vi "Display Continuous Probability Distributions.vi"() -> ()   [LabVIEW 2023]
doc: "This example VI uses Continuous PDF.vi, Continuous CDF.vi, Continuous Inverse CDF.vi to display continuous probability density functions, cumulative distribution functions, and inverse cumulative distribution functions for the beta, cauchy, chi-squared, exponential, gamma, laplace, and normal distributions."
uses:
  <vilib>/Analysis/1siggen.llb/Ramp Pattern by Samples.vi
  <vilib>/gmath/statdist.llb/Normal Moments.vi
  <vilib>/gmath/statdist.llb/Normal CDF.vi
  <vilib>/gmath/statdist.llb/Normal Inverse CDF.vi
  <vilib>/gmath/statdist.llb/Normal PDF.vi
  <vilib>/gmath/statdist.llb/Uniform CDF.vi
  <vilib>/gmath/statdist.llb/Uniform Inverse CDF.vi
  <vilib>/gmath/statdist.llb/Uniform PDF.vi
  <vilib>/gmath/statdist.llb/Uniform Moments.vi
  <vilib>/gmath/statdist.llb/Beta Moments.vi
  <vilib>/gmath/statdist.llb/Beta CDF.vi
  <vilib>/gmath/statdist.llb/Beta Inverse CDF.vi
  <vilib>/gmath/statdist.llb/Beta PDF.vi
  <vilib>/gmath/statdist.llb/Cauchy CDF.vi
  <vilib>/gmath/statdist.llb/Cauchy Inverse CDF.vi
  <vilib>/gmath/statdist.llb/Cauchy PDF.vi
  <vilib>/gmath/statdist.llb/Chi-Squared Moments.vi
  <vilib>/gmath/statdist.llb/Chi-Squared CDF.vi
  <vilib>/gmath/statdist.llb/Chi-Squared Inverse CDF.vi
  <vilib>/gmath/statdist.llb/Chi-Squared PDF.vi
  <vilib>/gmath/statdist.llb/Exp Moments.vi
  <vilib>/gmath/statdist.llb/Exp CDF.vi
  <vilib>/gmath/statdist.llb/Exp Inverse CDF.vi
  <vilib>/gmath/statdist.llb/Exp PDF.vi
  <vilib>/gmath/statdist.llb/Lognormal CDF.vi
  <vilib>/gmath/statdist.llb/Lognormal Inverse CDF.vi
  <vilib>/gmath/statdist.llb/Lognormal PDF.vi
  <vilib>/gmath/statdist.llb/Lognormal Moments.vi
  <vilib>/gmath/statdist.llb/Gamma Moments.vi
  <vilib>/gmath/statdist.llb/Gamma CDF.vi
  <vilib>/gmath/statdist.llb/Gamma Inverse CDF.vi
  <vilib>/gmath/statdist.llb/Gamma PDF.vi
  <vilib>/gmath/statdist.llb/Laplace Moments.vi
  <vilib>/gmath/statdist.llb/Laplace CDF.vi
  <vilib>/gmath/statdist.llb/Laplace Inverse CDF.vi
  <vilib>/gmath/statdist.llb/Laplace PDF.vi
  <vilib>/gmath/NI_Gmath.lvlib
  <vilib>/Analysis/NI_AALBase.lvlib
panel:
  in  "Stop":bool
  in  "Tab Control":T1(tab)
  in  "std (Normal)":dbl(slide)=4.0 min=0.0 scale=0.5..4.0
  in  "mean (Normal)":dbl(slide) scale=-5.0..5.0
  in  "end (Normal)":dbl=15.0
  in  "start (Normal)":dbl=-15.0
  in  "samples (Normal)":i32=200
  out "Variance (Normal)":dbl
  out "Mean (Normal)":dbl
  out "Normal Inverse Cumulative Distribution Function":cluster{dbl[], dbl[]}(graph)
  out "Normal Cumulative Distribution Function":cluster{"Ramp Pattern":dbl[], dbl[]}(graph)
  out "Normal Probability Density Function":cluster{"Ramp Pattern":dbl[], dbl[]}(graph)
  in  "x max":dbl(slide)=5.0 min=0.0 scale=0.0..5.0
  in  "x min":dbl(slide)=-5.0
  in  "end (Uniform)":dbl=10.0
  in  "start (Uniform)":dbl=-10.0
  in  "samples (Uniform)":i32=200
  out "Variance (Uniform)":dbl
  out "Mean (Uniform)":dbl
  out "Uniform Inverse Cumulative Distribution Function":cluster{dbl[], dbl[]}(graph)
  out "Uniform Cumulative Distribution Function":cluster{"Ramp Pattern":dbl[], dbl[]}(graph)
  out "Uniform Probability Density Function":cluster{"Ramp Pattern":dbl[], dbl[]}(graph)
  in  "start (Beta)":dbl min=0.0 max=1.0
  in  "end (Beta)":dbl=1.0 min=0.0 max=1.0
  in  "samples (Beta)":i32=100
  out "Variance (Beta)":dbl=0.031746031746031744
  out "Mean (Beta)":dbl=0.3333333333333333
  in  "b (Beta)":dbl(slide)=4.0 min=0.0 scale=0.1..100.0
  in  "a (Beta)":dbl(slide)=2.0 min=0.0 scale=0.1..10.0
  out "Beta Inverse Cumulative Distribution Function":cluster{dbl[], dbl[]}(graph)
  out "Beta Cumulative Distribution Function":cluster{"Ramp Pattern":dbl[], dbl[]}(graph)
  out "Beta Probability Density Function":cluster{"Ramp Pattern":dbl[], dbl[]}(graph)
  in  "end (Cauchy)":dbl=10.0
  in  "samples (Cauchy)":i32=100
  in  "start (Cauchy)":dbl=-10.0
  in  "b (Cauchy)":dbl(slide)=1.0 min=0.0 scale=0.1..10.0
  in  "a (Cauchy)":dbl(slide) scale=-10.0..10.0
  out "Cauchy Inverse Cumulative Distribution Function":cluster{dbl[], dbl[]}(graph)
  out "Cauchy Cumulative Distribution Function":cluster{"Ramp Pattern":dbl[], dbl[]}(graph)
  out "Cauchy Probability Density Function":cluster{"Ramp Pattern":dbl[], dbl[]}(graph)
  in  "end (Chi-Squared)":dbl=200.0
  in  "start (Chi-Squared)":dbl min=0.0
  in  "samples (Chi-Squared)":i32=200
  out "Variance (Chi-Squared)":dbl
  out "Mean (Chi-Squared)":dbl
  in  "degrees of freedom (k)":i32(slide)=80 min=1 scale=1.0..40.0
  out "Chi-Square Inverse Cumulative Distribution Function":cluster{dbl[], dbl[]}(graph)
  out "Chi-Square Cumulative Distribution Function":cluster{"Ramp Pattern":dbl[], dbl[]}(graph)
  out "Chi-Square Probability Density Function":cluster{"Ramp Pattern":dbl[], dbl[]}(graph)
  out "Exponential Cumulative Distribution Function":cluster{"Ramp Pattern":dbl[], dbl[]}(graph)
  in  "end (Exp)":dbl=15.0
  in  "start (Exp)":dbl min=0.0
  in  "samples (Exp)":i32=100
  out "Variance (Exp)":dbl
  out "Mean (Exp)":dbl
  in  "b (Exp)":dbl(slide)=4.0 min=0.0 scale=0.1..10.0
  in  "a (Exp)":dbl(slide) scale=0.0..10.0
  out "Exponential Inverse Cumulative Distribution Function":cluster{dbl[], dbl[]}(graph)
  out "Exponential Probability Density Function":cluster{"Ramp Pattern":dbl[], dbl[]}(graph)
  in  "location type":enum16{"mu - mean (log(X))", "median (X)"}(ring)
  in  "samples (Lognormal)":i32=200
  in  "mu or median (Lognormal)":dbl(slide)=1.0 scale=-5.0..5.0
  in  "start (Lognormal)":dbl
  in  "end (Lognormal)":dbl=10.0
  in  "std (Lognormal)":dbl(slide)=1.0 min=0.0 scale=0.5..4.0
  out "Variance (Lognormal)":dbl
  out "Mean (Lognormal)":dbl
  out "Lognormal Cumulative Distribution Function":cluster{"Ramp Pattern":dbl[], dbl[]}(graph)
  out "Lognormal Inverse Cumulative Distribution Function":cluster{dbl[], dbl[]}(graph)
  out "Lognormal PDF":cluster{"Ramp Pattern":dbl[], dbl[]}(graph)
  in  "end (Gamma)":dbl=100.0
  in  "start (Gamma)":dbl min=0.0
  in  "samples (Gamma)":i32=200
  out "Variance (Gamma)":dbl
  out "Mean (Gamma)":dbl
  in  "c (Gamma)":dbl(slide)=7.0 min=0.0 scale=0.1..10.0
  in  "b (Gamma)":dbl(slide)=3.0 min=0.0 scale=1.0..10.0
  out "Gamma Inverse Cumulative Distribution Function":cluster{dbl[], dbl[]}(graph)
  out "Gamma Cumulative Distribution Function":cluster{"Ramp Pattern":dbl[], dbl[]}(graph)
  out "Gamma Probability Density Function":cluster{"Ramp Pattern":dbl[], dbl[]}(graph)
  in  "end (Laplace)":dbl=15.0
  in  "start (Laplace)":dbl=-15.0
  in  "samples (Laplace)":i32=200
  in  "b (Laplace)":dbl(slide)=3.0 min=0.0 scale=0.0..10.0
  in  "a (Laplace)":dbl(slide) scale=-5.0..5.0
  out "Variance (Laplace)":dbl
  out "Mean (Laplace)":dbl
  out "Laplace Inverse Cumulative Distribution Function":cluster{dbl[], dbl[]}(graph)
  out "Laplace Cumulative Distribution Function":cluster{"Ramp Pattern":dbl[], dbl[]}(graph)
  out "Laplace Probability Density Function":cluster{"Ramp Pattern":dbl[], dbl[]}(graph)
  # "Overview: Demonstrates the use of the Continuous PDF VI, Continuous CDF VI, and Continuous Inverse CDF VI.\nInstructions:\n1. Run the VI.\n2. Switch between tabs to explore how the parameters affect each distribution.\n3. Click Stop to stop the VI."
  # "NOTE: According to theory, the Cauchy distribution does not have a moment generating function (mean and variance)"
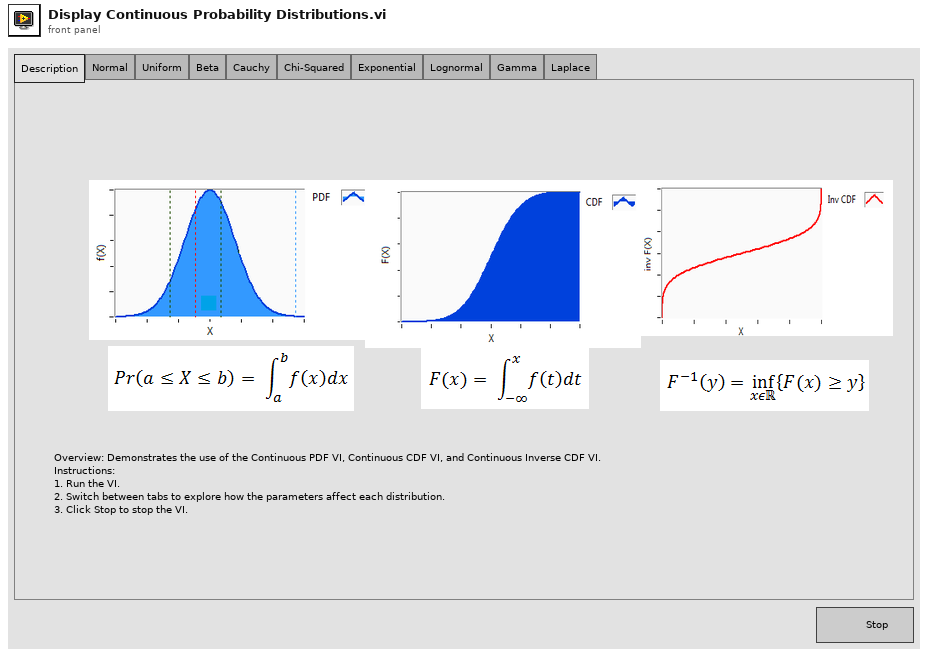
[diagram p1: front panel]
types:
  T1 = enum32{"Description", "Normal", "Uniform", "Beta", "Cauchy", "Chi-Squared", "Exponential", "Lognormal", "Gamma", "Laplace"}
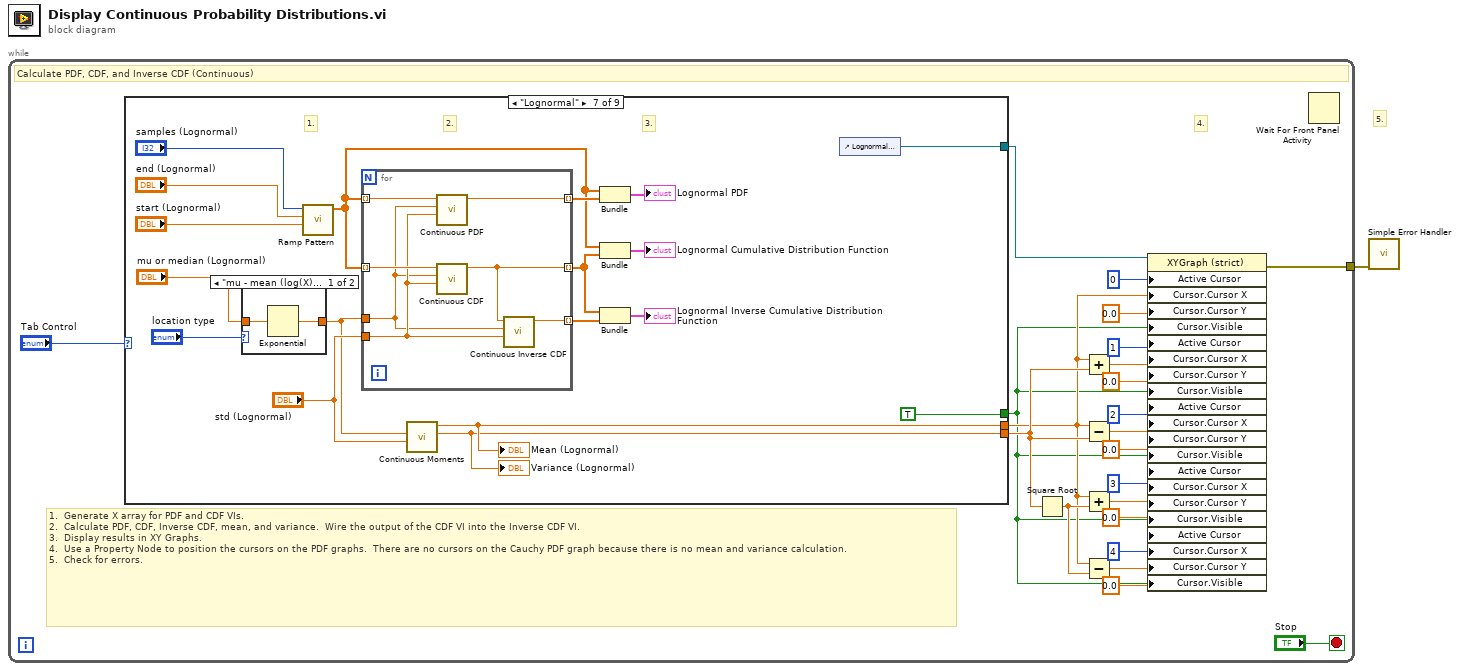
[diagram p0: block diagram]
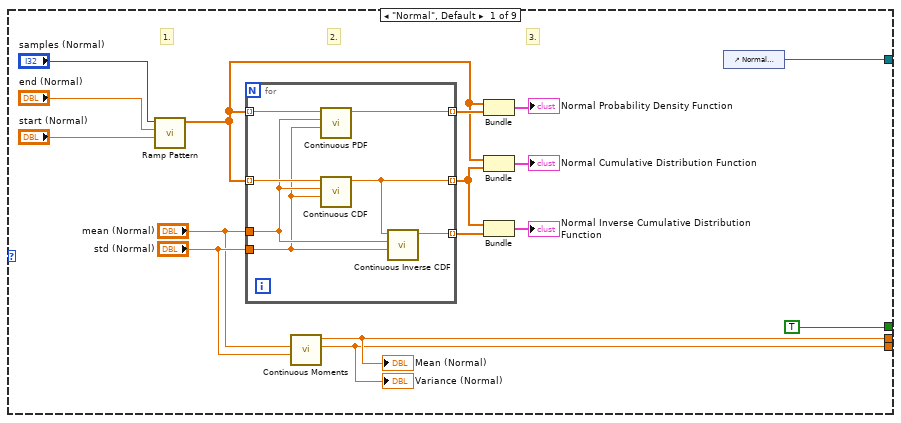
[diagram p2: hidden frame]
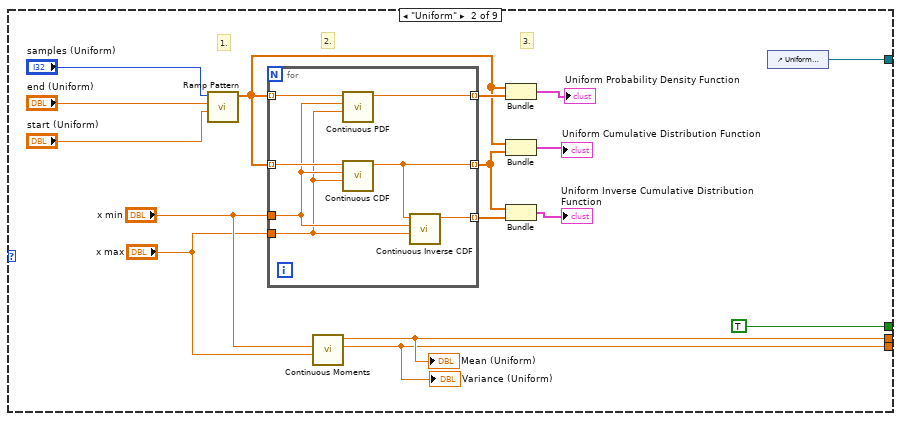
[diagram p3: hidden frame]
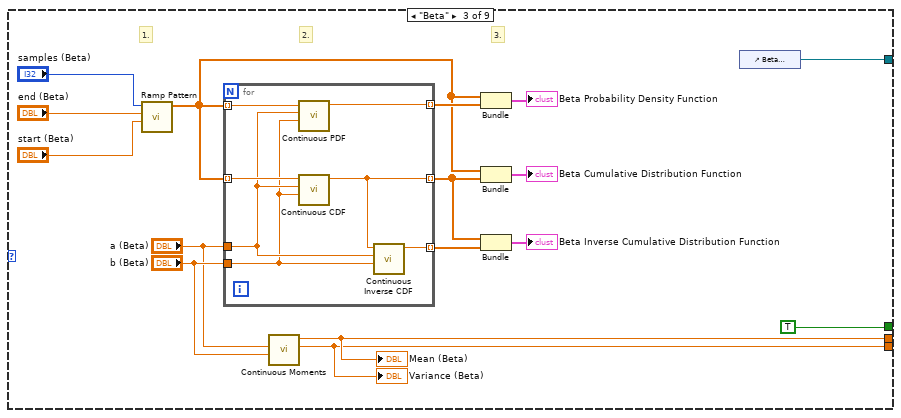
[diagram p4: hidden frame]
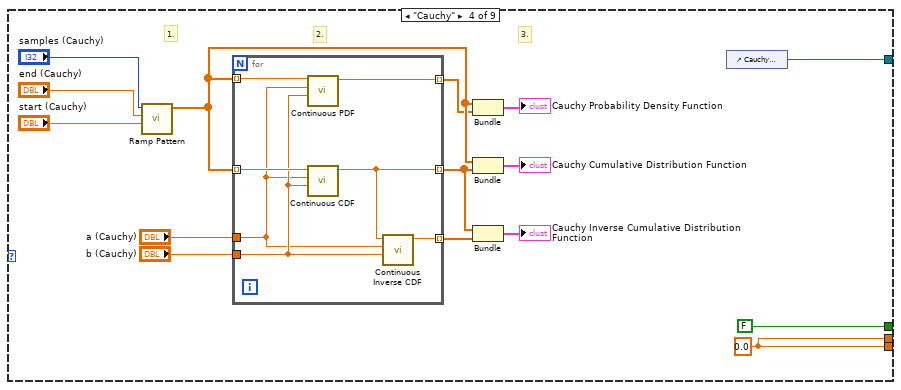
[diagram p5: hidden frame]
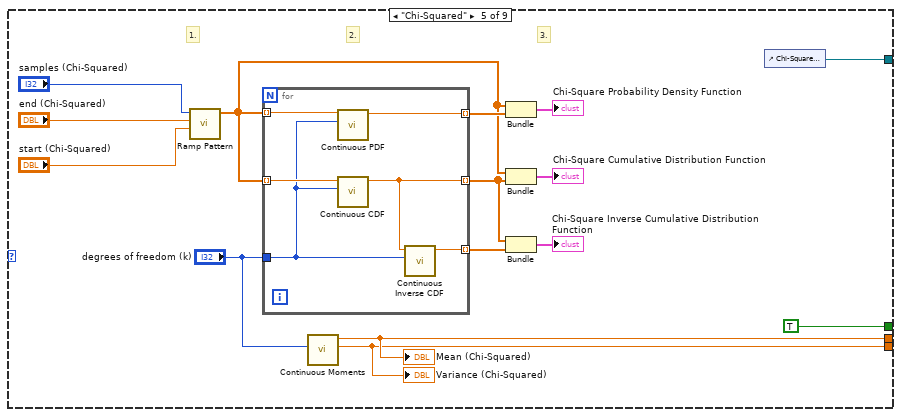
[diagram p6: hidden frame]
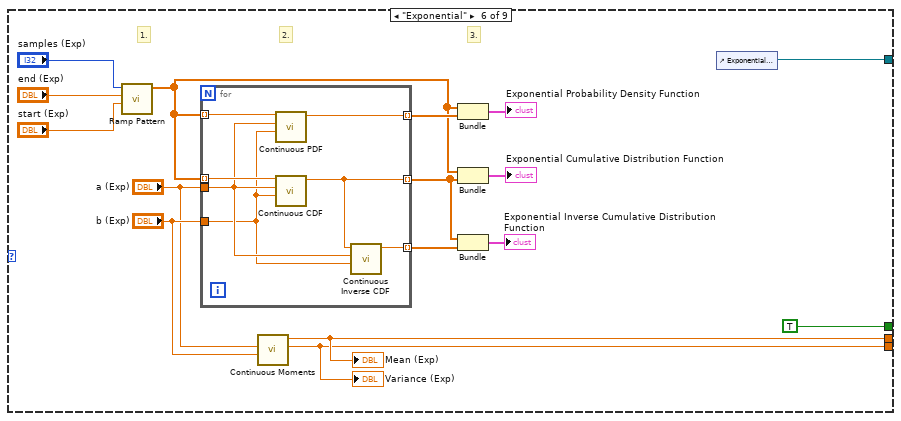
[diagram p7: hidden frame]
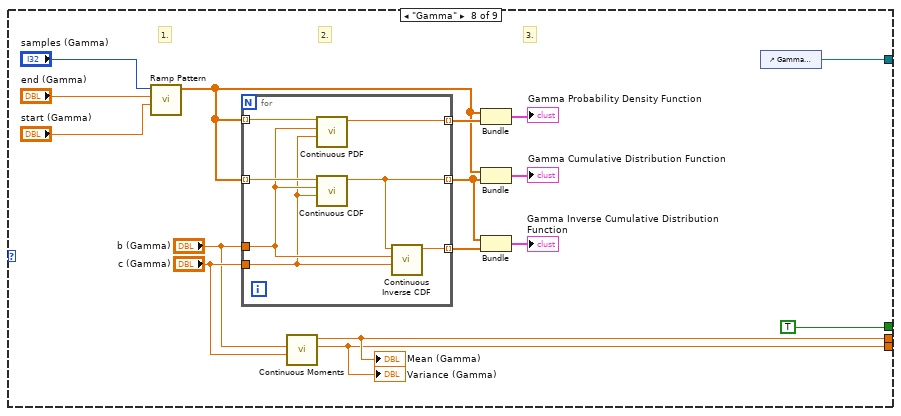
[diagram p9: hidden frame]
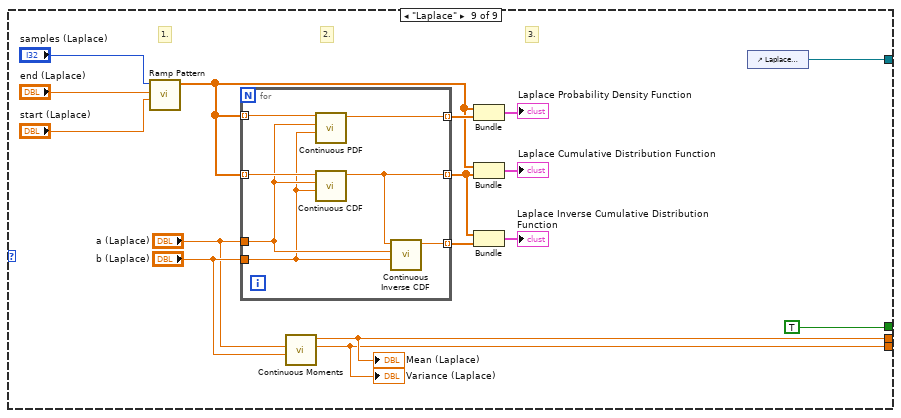
[diagram p10: hidden frame]
diagram:
  # "5."
  n1 = while {
    tunnel: [w5] -> w1
    stop <- "Stop" stop-if-true
    # "1.  Generate X array for PDF and CDF VIs.\n2.  Calculate PDF, CDF, Inverse CDF, mean, and variance.  Wire the output of the CDF VI into the Inverse CDF VI.  \n3.  Display results in XY Graphs.\n4.  Use a Property Node to position the cursors on the PDF graphs.  There are no cursors on the Cauchy PDF graph because there is no mean and variance calculation.\n5.  Check for errors."
    # "4."
    # "Calculate PDF, CDF, and Inverse CDF (Continuous)"
    n2 = case shown="\"Lognormal\"" "Tab Control" {
      tunnel: [w27 w53 w73 w94 w119 w139 w165 w190 w213] -> w4
      tunnel: [w26 w50 w72 w93 w118 w138 w164 w189 w212] -> w3
      tunnel: [w25 w49 w71 w93 w117 w137 w163 w188 w211] -> w10
      tunnel: [TRUE TRUE TRUE FALSE TRUE TRUE TRUE TRUE TRUE] -> w2
      frame "Normal", Default {
        # "3."
        # "2."
        # "1."
        n3 = call-poly <vilib>:"Ramp Pattern.vi"("start"="start (Normal)", "end"="end (Normal)", "samples"="samples (Normal)") -> ("Ramp Pattern"=w35:dbl[])  [unwired: 7 in, 1 out]
        n4 = for {
          tunnel: w35 -> [w46] mode=indexing
          tunnel: [w45] -> w36 mode=indexing
          tunnel: w35 -> [w44] mode=indexing
          tunnel: [w43] -> w33 mode=indexing
          tunnel: [w42] -> w34 mode=indexing
          tunnel: "mean (Normal)" -> [w41]
          tunnel: "std (Normal)" -> [w40]
          n5 = call-poly <vilib>:"Continuous PDF.vi"("std"=w40, "mean"=w41, "x"=w46) -> ("pdf(x)"=w45:dbl)  [unwired: 7 in, 1 out]
          n6 = call-poly <vilib>:"Continuous CDF.vi"("std"=w40, "mean"=w41, "x"=w44) -> ("cdf(x)"=w43:dbl)  [unwired: 7 in, 1 out]
          n7 = call-poly <vilib>:"Continuous Inverse CDF.vi"("std"=w40, "mean"=w41, "cdf(x)"=w43) -> ("x"=w42:dbl)  [unwired: 7 in, 1 out]
        }
        n8 = call-poly <vilib>:"Continuous Moments.vi"("std"="std (Normal)", "mean"="mean (Normal)") -> ("variance"=w25:dbl, "mean"=w26:dbl)  [unwired: 7 in, 1 out]
        "Mean (Normal)" <- w26
        "Variance (Normal)" <- w25
        n9 = Bundle("Ramp Pattern"=w35, w36) -> (→"Normal Probability Density Function":cluster{"Ramp Pattern":dbl[], dbl[]})  [unwired: 1 in]
        n10 = Bundle("Ramp Pattern"=w35, w33) -> (→"Normal Cumulative Distribution Function":cluster{"Ramp Pattern":dbl[], dbl[]})  [unwired: 1 in]
        n11 = Bundle(w33, w34) -> (→"Normal Inverse Cumulative Distribution Function":cluster{dbl[], dbl[]})  [unwired: 1 in]
        n12 = control-ref of="Normal Probability Density Function"() -> (w27:refnum<vi>)
      }
      frame "Uniform" {
        # "3."
        # "2."
        # "1."
        n13 = call-poly <vilib>:"Ramp Pattern.vi"("start"="start (Uniform)", "end"="end (Uniform)", "samples"="samples (Uniform)") -> ("Ramp Pattern"=w61:dbl[])  [unwired: 7 in, 1 out]
        n14 = for {
          tunnel: w61 -> [w69] mode=indexing
          tunnel: [w68] -> w62 mode=indexing
          tunnel: w61 -> [w67] mode=indexing
          tunnel: [w66] -> w59 mode=indexing
          tunnel: [w65] -> w60 mode=indexing
          tunnel: "x min" -> [w64]
          tunnel: "x max" -> [w63]
          n15 = call-poly <vilib>:"Continuous PDF.vi"("xmax"=w63, "xmin"=w64, "x"=w69) -> ("pdf(x)"=w68:dbl)  [unwired: 7 in, 1 out]
          n16 = call-poly <vilib>:"Continuous CDF.vi"("xmax"=w63, "xmin"=w64, "x"=w67) -> ("cdf(x)"=w66:dbl)  [unwired: 7 in, 1 out]
          n17 = call-poly <vilib>:"Continuous Inverse CDF.vi"("xmax"=w63, "xmin"=w64, "cdf(x)"=w66) -> ("x"=w65:dbl)  [unwired: 7 in, 1 out]
        }
        n18 = call-poly <vilib>:"Continuous Moments.vi"("xmax"="x max", "xmin"="x min") -> ("variance"=w49:dbl, "mean"=w50:dbl)  [unwired: 7 in, 1 out]
        "Mean (Uniform)" <- w50
        "Variance (Uniform)" <- w49
        n19 = Bundle("Ramp Pattern"=w61, w62) -> (→"Uniform Probability Density Function":cluster{"Ramp Pattern":dbl[], dbl[]})  [unwired: 1 in]
        n20 = Bundle("Ramp Pattern"=w61, w59) -> (→"Uniform Cumulative Distribution Function":cluster{"Ramp Pattern":dbl[], dbl[]})  [unwired: 1 in]
        n21 = Bundle(w59, w60) -> (→"Uniform Inverse Cumulative Distribution Function":cluster{dbl[], dbl[]})  [unwired: 1 in]
        n22 = control-ref of="Uniform Probability Density Function"() -> (w53:refnum<vi>)
      }
      frame "Beta" {
        # "3."
        # "2."
        # "1."
        n23 = call-poly <vilib>:"Ramp Pattern.vi"("start"="start (Beta)", "end"="end (Beta)", "samples"="samples (Beta)") -> ("Ramp Pattern"=w81:dbl[])  [unwired: 7 in, 1 out]
        n24 = for {
          tunnel: w81 -> [w92] mode=indexing
          tunnel: [w91] -> w82 mode=indexing
          tunnel: w81 -> [w90] mode=indexing
          tunnel: [w89] -> w79 mode=indexing
          tunnel: [w88] -> w80 mode=indexing
          tunnel: "a (Beta)" -> [w87]
          tunnel: "b (Beta)" -> [w86]
          n25 = call-poly <vilib>:"Continuous PDF.vi"("b"=w86, "a"=w87, "x"=w92) -> ("pdf(x)"=w91:dbl)  [unwired: 7 in, 1 out]
          n26 = call-poly <vilib>:"Continuous CDF.vi"("b"=w86, "a"=w87, "x"=w90) -> ("cdf(x)"=w89:dbl)  [unwired: 7 in, 1 out]
          n27 = call-poly <vilib>:"Continuous Inverse CDF.vi"("b"=w86, "a"=w87, "cdf(x)"=w89) -> ("x"=w88:dbl)  [unwired: 7 in, 1 out]
        }
        n28 = call-poly <vilib>:"Continuous Moments.vi"("b"="b (Beta)", "a"="a (Beta)") -> ("variance"=w71:dbl, "mean"=w72:dbl)  [unwired: 7 in, 1 out]
        "Mean (Beta)" <- w72
        "Variance (Beta)" <- w71
        n29 = Bundle("Ramp Pattern"=w81, w82) -> (→"Beta Probability Density Function":cluster{"Ramp Pattern":dbl[], dbl[]})  [unwired: 1 in]
        n30 = Bundle("Ramp Pattern"=w81, w79) -> (→"Beta Cumulative Distribution Function":cluster{"Ramp Pattern":dbl[], dbl[]})  [unwired: 1 in]
        n31 = Bundle(w79, w80) -> (→"Beta Inverse Cumulative Distribution Function":cluster{dbl[], dbl[]})  [unwired: 1 in]
        n32 = control-ref of="Beta Probability Density Function"() -> (w73:refnum<vi>)
      }
      frame "Cauchy" {
        w93 = 0.0
        # "3."
        # "2."
        # "1."
        n33 = call-poly <vilib>:"Ramp Pattern.vi"("start"="start (Cauchy)", "end"="end (Cauchy)", "samples"="samples (Cauchy)") -> ("Ramp Pattern"=w100:dbl[])  [unwired: 7 in, 1 out]
        n34 = for {
          tunnel: w100 -> [w114] mode=indexing
          tunnel: [w113] -> w99 mode=indexing
          tunnel: w100 -> [w112] mode=indexing
          tunnel: [w111] -> w104 mode=indexing
          tunnel: [w110] -> w105 mode=indexing
          tunnel: "a (Cauchy)" -> [w108]
          tunnel: "b (Cauchy)" -> [w109]
          n35 = call-poly <vilib>:"Continuous PDF.vi"("b"=w109, "a"=w108, "x"=w114) -> ("pdf(x)"=w113:dbl)  [unwired: 7 in, 1 out]
          n36 = call-poly <vilib>:"Continuous CDF.vi"("b"=w109, "a"=w108, "x"=w112) -> ("cdf(x)"=w111:dbl)  [unwired: 7 in, 1 out]
          n37 = call-poly <vilib>:"Continuous Inverse CDF.vi"("b"=w109, "a"=w108, "cdf(x)"=w111) -> ("x"=w110:dbl)  [unwired: 7 in, 1 out]
        }
        n38 = Bundle("Ramp Pattern"=w100, w99) -> (→"Cauchy Probability Density Function":cluster{"Ramp Pattern":dbl[], dbl[]})  [unwired: 1 in]
        n39 = Bundle("Ramp Pattern"=w100, w104) -> (→"Cauchy Cumulative Distribution Function":cluster{"Ramp Pattern":dbl[], dbl[]})  [unwired: 1 in]
        n40 = Bundle(w104, w105) -> (→"Cauchy Inverse Cumulative Distribution Function":cluster{dbl[], dbl[]})  [unwired: 1 in]
        n41 = control-ref of="Cauchy Probability Density Function"() -> (w94:refnum<vi>)
      }
      frame "Chi-Squared" {
        # "3."
        # "2."
        # "1."
        n42 = call-poly <vilib>:"Ramp Pattern.vi"("start"="start (Chi-Squared)", "end"="end (Chi-Squared)", "samples"="samples (Chi-Squared)") -> ("Ramp Pattern"=w126:dbl[])  [unwired: 7 in, 1 out]
        n43 = for {
          tunnel: w126 -> [w135] mode=indexing
          tunnel: [w134] -> w127 mode=indexing
          tunnel: w126 -> [w133] mode=indexing
          tunnel: [w132] -> w124 mode=indexing
          tunnel: [w131] -> w125 mode=indexing
          tunnel: "degrees of freedom (k)" -> [w130]
          n44 = call-poly <vilib>:"Continuous PDF.vi"("k"=w130, "x"=w135) -> ("pdf(x)"=w134:dbl)  [unwired: 8 in, 1 out]
          n45 = call-poly <vilib>:"Continuous CDF.vi"("k"=w130, "x"=w133) -> ("cdf(x)"=w132:dbl)  [unwired: 8 in, 1 out]
          n46 = call-poly <vilib>:"Continuous Inverse CDF.vi"("k"=w130, "cdf(x)"=w132) -> ("x"=w131:dbl)  [unwired: 8 in, 1 out]
        }
        n47 = call-poly <vilib>:"Continuous Moments.vi"("k"="degrees of freedom (k)") -> ("variance"=w117:dbl, "mean"=w118:dbl)  [unwired: 8 in, 1 out]
        "Mean (Chi-Squared)" <- w118
        "Variance (Chi-Squared)" <- w117
        n48 = Bundle("Ramp Pattern"=w126, w127) -> (→"Chi-Square Probability Density Function":cluster{"Ramp Pattern":dbl[], dbl[]})  [unwired: 1 in]
        n49 = Bundle("Ramp Pattern"=w126, w124) -> (→"Chi-Square Cumulative Distribution Function":cluster{"Ramp Pattern":dbl[], dbl[]})  [unwired: 1 in]
        n50 = Bundle(w124, w125) -> (→"Chi-Square Inverse Cumulative Distribution Function":cluster{dbl[], dbl[]})  [unwired: 1 in]
        n51 = control-ref of="Chi-Square Probability Density Function"() -> (w119:refnum<vi>)
      }
      frame "Exponential" {
        # "3."
        # "2."
        # "1."
        n52 = call-poly <vilib>:"Ramp Pattern.vi"("start"="start (Exp)", "end"="end (Exp)", "samples"="samples (Exp)") -> ("Ramp Pattern"=w147:dbl[])  [unwired: 7 in, 1 out]
        n53 = for {
          tunnel: w147 -> [w158] mode=indexing
          tunnel: [w157] -> w148 mode=indexing
          tunnel: w147 -> [w156] mode=indexing
          tunnel: [w155] -> w145 mode=indexing
          tunnel: [w154] -> w146 mode=indexing
          tunnel: "a (Exp)" -> [w153]
          tunnel: "b (Exp)" -> [w152]
          n54 = call-poly <vilib>:"Continuous PDF.vi"("b"=w152, "a"=w153, "x"=w158) -> ("pdf(x)"=w157:dbl)  [unwired: 7 in, 1 out]
          n55 = call-poly <vilib>:"Continuous CDF.vi"("b"=w152, "a"=w153, "x"=w156) -> ("cdf(x)"=w155:dbl)  [unwired: 7 in, 1 out]
          n56 = call-poly <vilib>:"Continuous Inverse CDF.vi"("b"=w152, "a"=w153, "cdf(x)"=w155) -> ("x"=w154:dbl)  [unwired: 7 in, 1 out]
        }
        n57 = call-poly <vilib>:"Continuous Moments.vi"("b"="b (Exp)", "a"="a (Exp)") -> ("variance"=w137:dbl, "mean"=w138:dbl)  [unwired: 7 in, 1 out]
        "Mean (Exp)" <- w138
        "Variance (Exp)" <- w137
        n58 = Bundle("Ramp Pattern"=w147, w148) -> (→"Exponential Probability Density Function":cluster{"Ramp Pattern":dbl[], dbl[]})  [unwired: 1 in]
        n59 = Bundle("Ramp Pattern"=w147, w145) -> (→"Exponential Cumulative Distribution Function":cluster{"Ramp Pattern":dbl[], dbl[]})  [unwired: 1 in]
        n60 = Bundle(w145, w146) -> (→"Exponential Inverse Cumulative Distribution Function":cluster{dbl[], dbl[]})  [unwired: 1 in]
        n61 = control-ref of="Exponential Probability Density Function"() -> (w139:refnum<vi>)
      }
      frame "Lognormal" {
        # "3."
        # "2."
        # "1."
        n62 = case shown="\"mu - mean (log(X))\", Default" "location type" {
          tunnel: "mu or median (Lognormal)" -> [w178 w179]
          tunnel: [w177 w179] -> w160
          frame "mu - mean (log(X))", Default {
            n63 = Exponential(1:w178) -> (0:w177:dbl)
          }
          frame "median (X)" {
          }
        }
        n64 = call-poly <vilib>:"Ramp Pattern.vi"("start"="start (Lognormal)", "end"="end (Lognormal)", "samples"="samples (Lognormal)") -> ("Ramp Pattern"=w172:dbl[])  [unwired: 7 in, 1 out]
        n65 = for {
          tunnel: w172 -> [w186] mode=indexing
          tunnel: [w185] -> w173 mode=indexing
          tunnel: w172 -> [w184] mode=indexing
          tunnel: [w183] -> w170 mode=indexing
          tunnel: [w182] -> w171 mode=indexing
          tunnel: w160 -> [w180]
          tunnel: "std (Lognormal)" -> [w181]
          n66 = call-poly <vilib>:"Continuous PDF.vi"("c"=w181, "b"=w180, "x"=w186) -> ("pdf(x)"=w185:dbl)  [unwired: 7 in, 1 out]
          n67 = call-poly <vilib>:"Continuous CDF.vi"("c"=w181, "b"=w180, "x"=w184) -> ("cdf(x)"=w183:dbl)  [unwired: 7 in, 1 out]
          n68 = call-poly <vilib>:"Continuous Inverse CDF.vi"("c"=w181, "b"=w180, "cdf(x)"=w183) -> ("x"=w182:dbl)  [unwired: 7 in, 1 out]
        }
        n69 = call-poly <vilib>:"Continuous Moments.vi"("c"="std (Lognormal)", "b"=w160) -> ("variance"=w163:dbl, "mean"=w164:dbl)  [unwired: 7 in, 1 out]
        "Mean (Lognormal)" <- w164
        "Variance (Lognormal)" <- w163
        n70 = Bundle("Ramp Pattern"=w172, w173) -> (→"Lognormal PDF":cluster{"Ramp Pattern":dbl[], dbl[]})  [unwired: 1 in]
        n71 = Bundle("Ramp Pattern"=w172, w170) -> (→"Lognormal Cumulative Distribution Function":cluster{"Ramp Pattern":dbl[], dbl[]})  [unwired: 1 in]
        n72 = Bundle(w170, w171) -> (→"Lognormal Inverse Cumulative Distribution Function":cluster{dbl[], dbl[]})  [unwired: 1 in]
        n73 = control-ref of="Lognormal PDF"() -> (w165:refnum<vi>)
      }
      frame "Gamma" {
        # "3."
        # "2."
        # "1."
        n74 = call-poly <vilib>:"Ramp Pattern.vi"("start"="start (Gamma)", "end"="end (Gamma)", "samples"="samples (Gamma)") -> ("Ramp Pattern"=w198:dbl[])  [unwired: 7 in, 1 out]
        n75 = for {
          tunnel: w198 -> [w209] mode=indexing
          tunnel: [w208] -> w199 mode=indexing
          tunnel: w198 -> [w207] mode=indexing
          tunnel: [w206] -> w196 mode=indexing
          tunnel: [w205] -> w197 mode=indexing
          tunnel: "b (Gamma)" -> [w204]
          tunnel: "c (Gamma)" -> [w203]
          n76 = call-poly <vilib>:"Continuous PDF.vi"("c"=w203, "b"=w204, "x"=w209) -> ("pdf(x)"=w208:dbl)  [unwired: 7 in, 1 out]
          n77 = call-poly <vilib>:"Continuous CDF.vi"("c"=w203, "b"=w204, "x"=w207) -> ("cdf(x)"=w206:dbl)  [unwired: 7 in, 1 out]
          n78 = call-poly <vilib>:"Continuous Inverse CDF.vi"("c"=w203, "b"=w204, "cdf(x)"=w206) -> ("x"=w205:dbl)  [unwired: 7 in, 1 out]
        }
        n79 = call-poly <vilib>:"Continuous Moments.vi"("c"="c (Gamma)", "b"="b (Gamma)") -> ("variance"=w188:dbl, "mean"=w189:dbl)  [unwired: 7 in, 1 out]
        "Mean (Gamma)" <- w189
        "Variance (Gamma)" <- w188
        n80 = Bundle("Ramp Pattern"=w198, w199) -> (→"Gamma Probability Density Function":cluster{"Ramp Pattern":dbl[], dbl[]})  [unwired: 1 in]
        n81 = Bundle("Ramp Pattern"=w198, w196) -> (→"Gamma Cumulative Distribution Function":cluster{"Ramp Pattern":dbl[], dbl[]})  [unwired: 1 in]
        n82 = Bundle(w196, w197) -> (→"Gamma Inverse Cumulative Distribution Function":cluster{dbl[], dbl[]})  [unwired: 1 in]
        n83 = control-ref of="Gamma Probability Density Function"() -> (w190:refnum<vi>)
      }
      frame "Laplace" {
        # "3."
        # "2."
        # "1."
        n84 = call-poly <vilib>:"Ramp Pattern.vi"("start"="start (Laplace)", "end"="end (Laplace)", "samples"="samples (Laplace)") -> ("Ramp Pattern"=w221:dbl[])  [unwired: 7 in, 1 out]
        n85 = for {
          tunnel: w221 -> [w232] mode=indexing
          tunnel: [w231] -> w222 mode=indexing
          tunnel: w221 -> [w230] mode=indexing
          tunnel: [w229] -> w219 mode=indexing
          tunnel: [w228] -> w220 mode=indexing
          tunnel: "a (Laplace)" -> [w227]
          tunnel: "b (Laplace)" -> [w226]
          n86 = call-poly <vilib>:"Continuous PDF.vi"("b"=w226, "a"=w227, "x"=w232) -> ("pdf(x)"=w231:dbl)  [unwired: 7 in, 1 out]
          n87 = call-poly <vilib>:"Continuous CDF.vi"("b"=w226, "a"=w227, "x"=w230) -> ("cdf(x)"=w229:dbl)  [unwired: 7 in, 1 out]
          n88 = call-poly <vilib>:"Continuous Inverse CDF.vi"("b"=w226, "a"=w227, "cdf(x)"=w229) -> ("x"=w228:dbl)  [unwired: 7 in, 1 out]
        }
        n89 = call-poly <vilib>:"Continuous Moments.vi"("b"="b (Laplace)", "a"="a (Laplace)") -> ("variance"=w211:dbl, "mean"=w212:dbl)  [unwired: 7 in, 1 out]
        "Mean (Laplace)" <- w212
        "Variance (Laplace)" <- w211
        n90 = Bundle("Ramp Pattern"=w221, w222) -> (→"Laplace Probability Density Function":cluster{"Ramp Pattern":dbl[], dbl[]})  [unwired: 1 in]
        n91 = Bundle("Ramp Pattern"=w221, w219) -> (→"Laplace Cumulative Distribution Function":cluster{"Ramp Pattern":dbl[], dbl[]})  [unwired: 1 in]
        n92 = Bundle(w219, w220) -> (→"Laplace Inverse Cumulative Distribution Function":cluster{dbl[], dbl[]})  [unwired: 1 in]
        n93 = control-ref of="Laplace Probability Density Function"() -> (w213:refnum<vi>)
      }
    }
    n94 = Square Root(x=w10) -> (sqrt(x)=w8:dbl)
    n95 = Add(x=w3, y=w10) -> (x+y=w12:dbl)
    n96 = Subtract(x=w3, y=w10) -> (x-y=w11:dbl)
    n97 = Add(x=w3, y=w8) -> (x+y=w9:dbl)
    n98 = Subtract(x=w3, y=w8) -> (x-y=w7:dbl)
    n99 = property on="Property Node" class="XYGraph (strict)"(reference=w4, "Active Cursor"=u32 0, "Cursor.Cursor X"=w3, "Cursor.Cursor Y"=0.0 ("Cursor.Cursor Position:Cursor Y"), "Cursor.Visible"=w2, "Active Cursor"=u32 1, "Cursor.Cursor X"=w12, "Cursor.Cursor Y"=0.0 ("Cursor.Cursor Position:Cursor Y"), "Cursor.Visible"=w2, "Active Cursor"=u32 2, "Cursor.Cursor X"=w11, "Cursor.Cursor Y"=0.0 ("Cursor.Cursor Position:Cursor Y"), "Cursor.Visible"=w2, "Active Cursor"=u32 3, "Cursor.Cursor X"=w9, "Cursor.Cursor Y"=0.0 ("Cursor.Cursor Position:Cursor Y"), "Cursor.Visible"=w2, "Active Cursor"=u32 4, "Cursor.Cursor X"=w7, "Cursor.Cursor Y"=0.0 ("Cursor.Cursor Position:Cursor Y"), "Cursor.Visible"=w2) -> (error out=w5:errorcluster)  [unwired: 1 in, 1 out]
    n100 = Wait For Front Panel Activity() -> ()  [unwired: 3 in, 1 out]
  }
  n101 = call <vilib>:"Simple Error Handler.vi"("error in (no error)"=w1) -> ()  [unwired: 4 in, 5 out]
